vi "Untitled 12.vi"(8 "error in (no error)":errorcluster, 11 "FlatSequenceFrame in":refnum<vi>) -> (0 "error out":errorcluster, 3 "FlatSequenceFrame out":refnum<vi>)   [LabVIEW 2011]
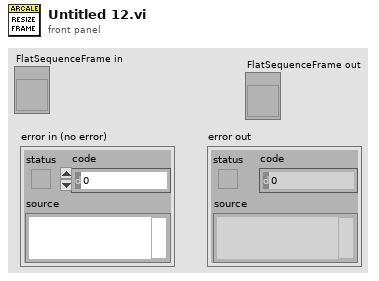
[diagram p1: front panel]
types:
  T1 = typedef "LVRectTypeDef.ctl" = cluster{"left":i16, "top":i16, "right":i16, "bottom":i16}
  T2 = typedef "LVBoundsTypeDef.ctl" = cluster{"Width":u32, "Height":u32}
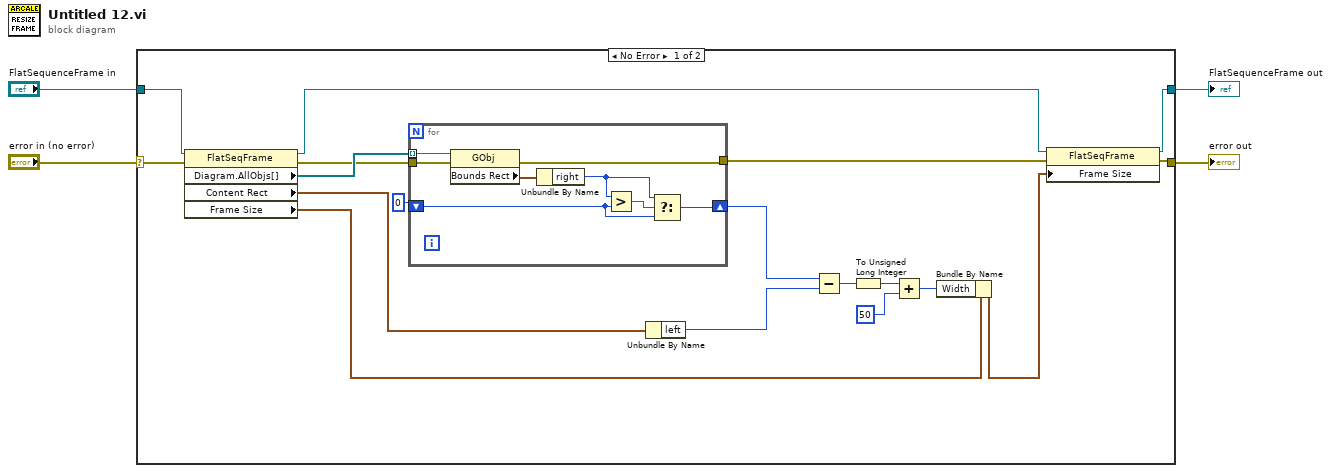
[diagram p0: block diagram]
diagram:
  n1 = case shown="No Error" "error in (no error)" {
    selector: "error in (no error)" -> [w6 w32]
    tunnel: "FlatSequenceFrame in" -> [w22 w31]
    tunnel: [w7 w31] -> w3
    tunnel: [w5 w32] -> w1
    frame No Error {
      n2 = property class="FlatSeqFrame"(reference=w22, error in=w6) -> (reference out=w19:refnum<vi>, error out=w15:errorcluster, "Diagram.AllObjs[]"=w21:refnum<vi>[], "Content Rect"=w20:T1, "Frame Size"=w18:T2)
      n3 = for {
        tunnel: w21 -> [w30] mode=indexing
        shift-right: [w27] -> w13
        shift-left: i16 0 ("right") -> [w25]
        tunnel: w15 -> [w24]
        tunnel: [w23] -> w14
        n4 = property class="GObj"(reference=w30, error in=w24) -> (error out=w23:errorcluster, "Bounds Rect"=w29:T1)  [unwired: 1 out]
        n5 = Unbundle By Name(w29) -> ("right"=w26:i16)
        n6 = Greater?(x=w26, y=w25) -> (0:w28:bool)
        n7 = Select(t=w26, s=w28, f=w25) -> (s? t:f=w27:i16)
      }
      n8 = Unbundle By Name(w20) -> ("left"=w12:i16)
      n9 = Subtract(x=w13, y=w12) -> (x-y=w11:i16)
      n10 = To Unsigned Long Integer(number=w11) -> (unsigned 32bit integer=w10:u32)
      n11 = Add(x=w10, y=u32 50) -> (x+y=w8:u32)
      n12 = Bundle By Name(cluster=w18, "Width"=w8) -> (w17:T2)
      n13 = property class="FlatSeqFrame"(reference=w19, error in=w14, "Frame Size"=w17) -> (reference out=w7:refnum<vi>, error out=w5:errorcluster)
    }
    frame Error {
    }
  }
  "FlatSequenceFrame out" <- w3
  "error out" <- w1
